vi "3.7 .vi"() -> ()   [LabVIEW 2019]
panel:
  out "hoeveel keer tot 5":dbl
  out "Numeric":dbl
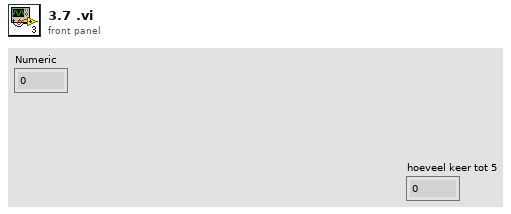
[diagram p1: front panel]
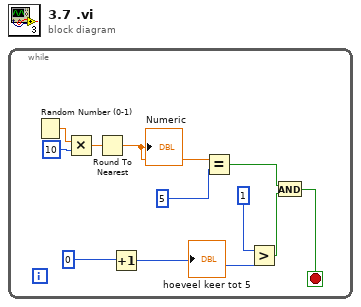
[diagram p0: block diagram]
diagram:
  n1 = while {
    stop <- w4 stop-if-true
    n2 = Random Number (0-1)() -> (number: 0 to 1=w11:dbl)
    n3 = Multiply(x=w11, y=10) -> (x*y=w9:dbl)
    n4 = Round To Nearest(number=w9) -> (nearest integer value=w7:dbl)
    "Numeric" <- w7
    n5 = Increment(x=0) -> (x+1=w3:i32)
    "hoeveel keer tot 5" <- w3
    n6 = Equal?(x=w7, y=5) -> (x = y?=w5:bool)
    n7 = Greater?(x=1, y=w3) -> (0:w2:bool)
    n8 = And(x=w5, y=w2) -> (x .and. y?=w4:bool)
  }
